vi "fgv.vi"(7 "Command":T1, 8 "error in (no error)":errorcluster, 10 "Car Position Slider":u8(slide) max=3 scale=0.0..4.0) -> (0 "error out":errorcluster, 2 "Car Position Slider 2":u8(slide) max=3 scale=0.0..4.0)   [LabVIEW 2013]
uses:
  fgv.ctl
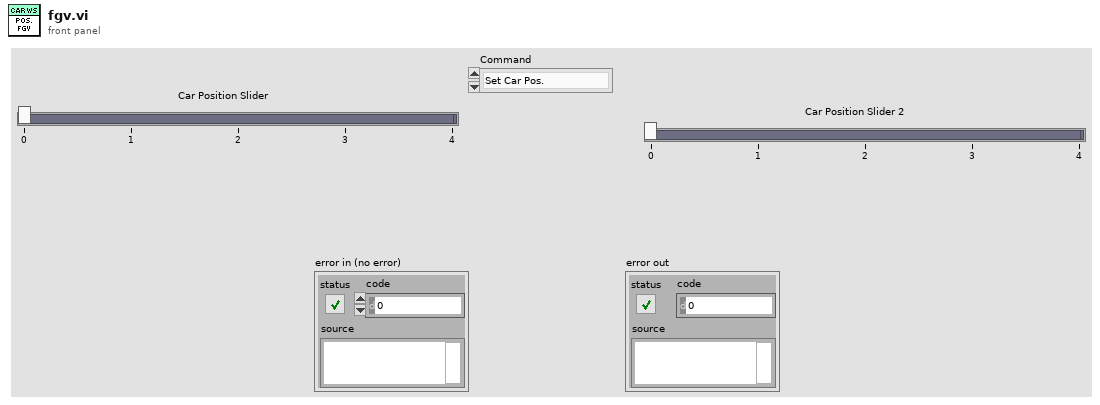
[diagram p1: front panel]
types:
  T1 = typedef "fgv.ctl" = enum16{"Set Car Pos.", "Get Car Pos."}
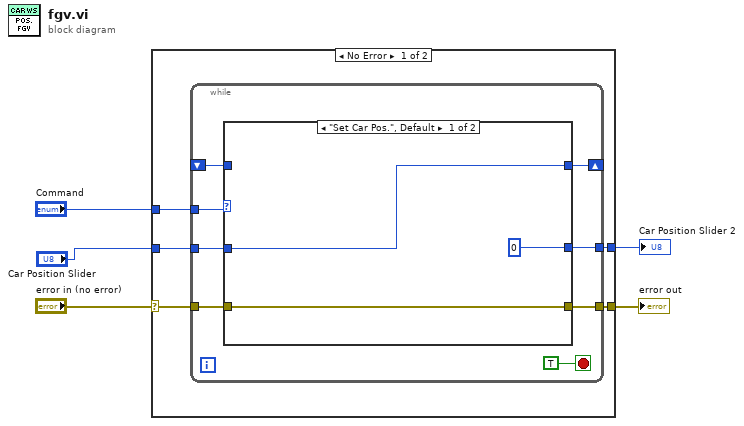
[diagram p0: block diagram]
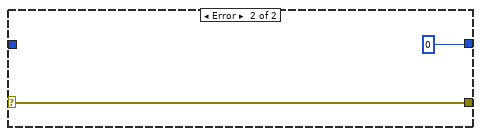
[diagram p3: hidden frame]
diagram:
  n1 = case shown="No Error" "error in (no error)" {
    selector: "error in (no error)" -> [w6 w25]
    tunnel: "Command" -> [w10 _]
    tunnel: "Car Position Slider" -> [w9 _]
    tunnel: [w8 u8 0 ("Numeric out")] -> w1
    tunnel: [w7 w25] -> w5
    frame No Error {
      n2 = while {
        tunnel: w10 -> [w17]
        tunnel: w9 -> [w16]
        shift-right: [w15] -> _
        shift-left: _ -> [w14]
        tunnel: [w13] -> w8
        tunnel: [w12] -> w7
        tunnel: w6 -> [w11]
        stop <- TRUE stop-if-true
        n3 = case shown="\"Set Car Pos.\", Default" w17 {
          tunnel: w16 -> [w21 _]
          tunnel: [w21 w23] -> w15
          tunnel: w14 -> [_ w23]
          tunnel: [u8 0 ("Numeric out") w23] -> w13
          tunnel: [w20 w22] -> w12
          tunnel: w11 -> [w20 w22]
          frame "Set Car Pos.", Default {
          }
          frame "Get Car Pos." {
          }
        }
      }
    }
    frame Error {
    }
  }
  "error out" <- w5
  "Car Position Slider 2" <- w1
